vi "Open PG.vi"(8 "error in (no error)":errorcluster, 11 "Data.PG in":refnum<class "Data.PGSQL.lvclass">) -> (0 "error out":errorcluster, 3 "Data.PG out":refnum<class "Data.PGSQL.lvclass">)   [LabVIEW 2013, in "Data.PGSQL.lvclass"]
uses:
  Data.PGSQL.lvclass
  Data.PGSQL.lvclass/Data.PGSQL.ctl
  PostgreSQL Library/Connection/PQ Connection.lvclass
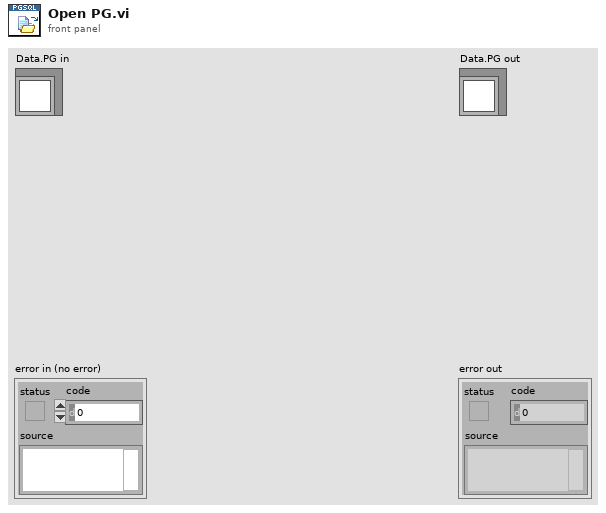
[diagram p1: front panel]
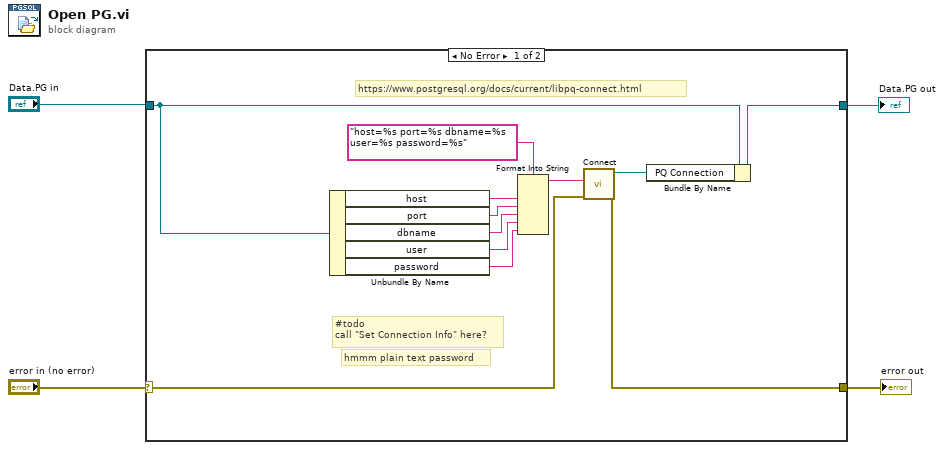
[diagram p0: block diagram]
diagram:
  n1 = case shown="No Error" "error in (no error)" {
    selector: "error in (no error)" -> [w15 w18]
    tunnel: [w11 w18] -> w2
    tunnel: "Data.PG in" -> [w5 w17]
    tunnel: [w16 w17] -> w1
    frame No Error {
      # "#todo\ncall \"Set Connection Info\" here?"
      # "hmmm plain text password"
      # "https://www.postgresql.org/docs/current/libpq-connect.html"
      n2 = Unbundle By Name(w5) -> ("host"=w10:string, "port"=w9:string, "dbname"=w8:string, "user"=w7:string, "password"=w6:string)
      n3 = Format Into String(format string="host=%s port=%s dbname=%s user=%s password=%s", w10, w9, w8, w7, w6) -> (resulting string=w12:string)  [unwired: 2 in, 1 out]
      n4 = call "Connect.vi"("error in (no error)"=w15, "Connection Strings"=w12) -> ("error out"=w11:errorcluster, "PQ Connection out"=w14:refnum<class "PQ Connection.lvclass">)  [unwired: 8 in]
      n5 = Bundle By Name(cluster=w5, "PQ Connection"=w14) -> (w16:refnum<class "Data.PGSQL.lvclass">)
    }
    frame Error {
    }
  }
  "error out" <- w2
  "Data.PG out" <- w1
